vi "Remove Embedded Data Logger Custom Device.vi"(8 "error in":errorcluster, 11 "embedded data logger custom device":T1=18446744073709551615 format="%.0x") -> (0 "error out":errorcluster)   [LabVIEW 2027, in "Embedded Data Logger Scripting.lvlib"]
uses:
  Embedded Data Logger Scripting.lvlib
  <vilib>/NI VeriStand/Custom Device API/Custom Device Item Ref.ctl
  <vilib>/NI VeriStand/Custom Device API/Custom Device API.lvlib
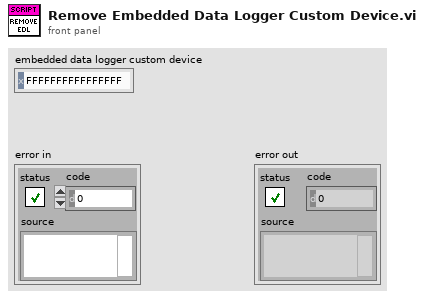
[diagram p1: front panel]
types:
  T1 = typedef "Custom Device API.lvlib/Custom Device Item Ref.ctl" = u64
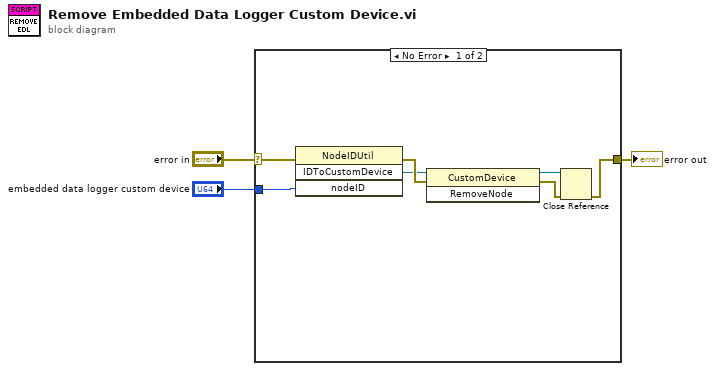
[diagram p0: block diagram]
diagram:
  n1 = case shown="No Error" "error in" {
    selector: "error in" -> [w10 w11]
    tunnel: [w5 w11] -> w2
    tunnel: "embedded data logger custom device" -> [w9 _]
    frame No Error {
      n2 = invoke class="NodeIDUtil" method="IDToCustomDevice"(error in=w10, "nodeID"=w9) -> (error out=w8:errorcluster, "IDToCustomDevice"=w6:refnum<k39>)  [unwired: 2 in, 2 out]
      n3 = invoke class="CustomDevice" method="RemoveNode"(reference=w6, error in=w8) -> (reference out=w4:refnum<k39>, error out=w7:errorcluster)  [unwired: 1 in, 1 out]
      n4 = Close Reference(reference=w4, error in (no error)=w7) -> (error out=w5:errorcluster)
    }
    frame Error {
    }
  }
  "error out" <- w2
